vi "API - Add System Mappings.vi"(8 "error in (no error)":errorcluster, 10 "Channels":T1[](array[typedef]) {"Destination Ref" format="%.0x"}, 11 "Rx Section Ref In":T2 format="%.0x") -> (0 "error out":errorcluster, 3 "Rx Section Ref Out":T2 format="%.0x")   [LabVIEW 2016, in "UDP-Custom-Device System Explorer.lvlib"]
uses:
  UDP-Custom-Device System Explorer.lvlib
  <vilib>/NI Veristand/Custom Device API/Custom Device Item Ref.ctl
  TypeDef - Channel Data.ctl
  Shared/DataTypes.ctl
  NationalInstruments.VeriStand.SystemDefinitionAPI
  <vilib>/NI Veristand/Custom Device Tools/Custom Device Utility Library/NI VeriStand - Search for Item by Name.vi
  <vilib>/NI VeriStand/Custom Device API/Custom Device API.lvlib
  <vilib>/NI VeriStand/Custom Device Tools/Custom Device Utility Library/Custom Device Utility Library.lvlib
  Shared/UDP-Custom-Device Shared.lvlib
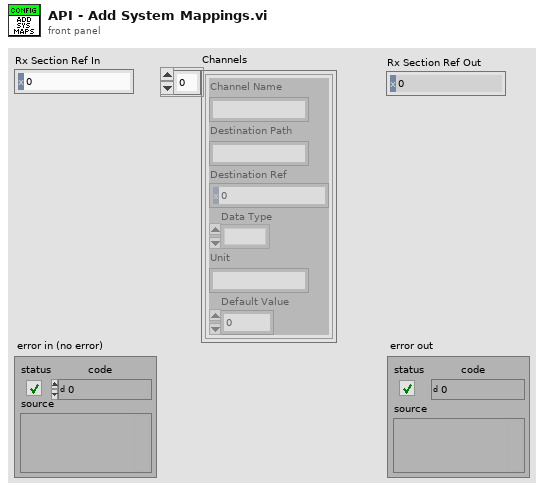
[diagram p1: front panel]
types:
  T1 = typedef "UDP-Custom-Device System Explorer.lvlib/TypeDef - Channel Data.ctl" = cluster{"Channel Name":string, "Destination Path":string, "Destination Ref":T2, "Data Type":T3, "Unit":string, "Default Value":dbl}
  T2 = typedef "Custom Device API.lvlib/Custom Device Item Ref.ctl" = u64
  T3 = typedef "UDP-Custom-Device Shared.lvlib/DataTypes.ctl" = enum16{""}
  T4 = typedef "Custom Device API.lvlib/Custom Device Pointer.ctl" = refnum<k24>
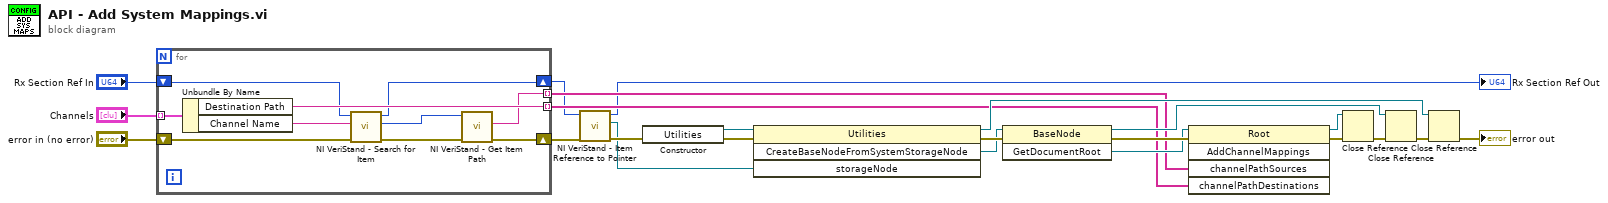
[diagram p0: block diagram]
diagram:
  n1 = for {
    tunnel: "Channels" -> [w33] mode=indexing
    tunnel: [w32] -> w5 mode=indexing
    shift-right: [w26] -> w4
    shift-left: "error in (no error)" -> [w30]
    shift-right: [w28] -> w3
    shift-left: "Rx Section Ref In" -> [w29]
    tunnel: [w24] -> w6 mode=indexing
    n2 = Unbundle By Name(w33) -> ("Destination Path"=w32:string, "Channel Name"=w31:string)
    n3 = call-poly <vilib>:"NI VeriStand - Search for Item.vi"("error in"=w30, "Item Name"=w31, "Section Ref in"=w29) -> ("error out"=w27:errorcluster, "Item Ref"=w25:T2, "Section Ref out"=w28:T2)  [unwired: 5 in, 1 out]
    n4 = call <vilib>:"NI VeriStand - Get Item Path.vi"("error in (no error)"=w27, "Item Ref in"=w25) -> ("error out"=w26:errorcluster, "Path"=w24:string)  [unwired: 6 in, 2 out]
  }
  n5 = call <vilib>:"NI VeriStand - Item Reference to Pointer.vi"("error in (no error)"=w4, "Item Ref in"=w3) -> ("error out"=w12:errorcluster, "Node Pointer"=w11:T4, "Item Ref out"=→"Rx Section Ref Out":T2)  [unwired: 6 in, 1 out]
  n6 = constructor class="Utilities"(error in=w12) -> (reference out=w1:refnum<k24>, error out=w15:errorcluster)  [unwired: 2 in, 1 out]
  n7 = invoke class="Utilities" method="CreateBaseNodeFromSystemStorageNode"(reference=w1, error in=w15, "storageNode"=w11) -> (reference out=w13:refnum<k24>, error out=w18:errorcluster, "CreateBaseNodeFromSystemStorageNode"=w16:refnum<k24>)  [unwired: 1 in, 1 out]
  n8 = invoke class="BaseNode" method="GetDocumentRoot"(reference=w16, error in=w18) -> (reference out=w14:refnum<k24>, error out=w19:errorcluster, "GetDocumentRoot"=w17:refnum<k24>)  [unwired: 1 in]
  n9 = invoke class="Root" method="AddChannelMappings"(reference=w17, error in=w19, "channelPathSources"=w6, "channelPathDestinations"=w5) -> (reference out=w21:refnum<k24>, error out=w20:errorcluster)  [unwired: 1 in, 3 out]
  n10 = Close Reference(reference=w21, error in (no error)=w20) -> (error out=w22:errorcluster)
  n11 = Close Reference(reference=w14, error in (no error)=w22) -> (error out=w23:errorcluster)
  n12 = Close Reference(reference=w13, error in (no error)=w23) -> (error out=→"error out":errorcluster)
